vi "Pre Launch Init.vi"(11 "Sensor in":refnum<class "Sensor.lvclass">) -> (0 "error out":errorcluster, 3 "Sensor out":refnum<class "Sensor.lvclass">)   [LabVIEW 2018, in "Sensor.lvlib" / "Sensor.lvclass"]
doc: "Sends a high priority message to it's self to notify the monitor that it's spawned. If it's in the runtime environment, this message is never sent, meaning the monitor will never spawn\n\nCopyright: MGI\nAuthored by: Derek Trepanier"
uses:
  Sensor.lvclass
  Sensor.lvclass/Sensor.ctl
  Actor Monitor/Actor/Monitored Actor.lvclass
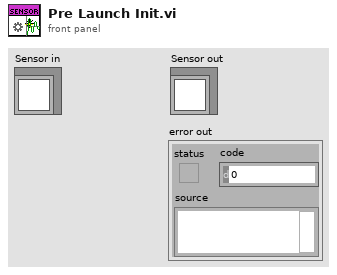
[diagram p1: front panel]
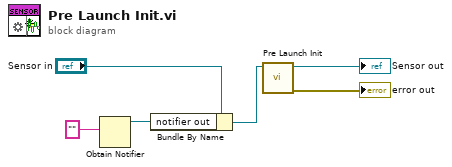
[diagram p0: block diagram]
diagram:
  n1 = Obtain Notifier(notification data type="") -> (notifier out=w4:refnum<notifier>)  [unwired: 3 in, 2 out]
  n2 = Bundle By Name(cluster="Sensor in", "notifier out"=w4) -> (w1:refnum<class "Sensor.lvclass">)
  n3 = call-parent "Pre Launch Init.vi"("Monitored Actor in"=w1) -> ("error out"=→"error out":errorcluster, "Monitored Actor out"=→"Sensor out":refnum<class "Sensor.lvclass">)  [unwired: 9 in]
